vi "PicoScope5000aGetRapidBlockBulk.vi"(0 "handle in":i16, 1 "Rapid Block Acquisition Settings":T4, 2 "Buffer and Transfer Settings":T3 {"Down-Sample Mode" items=["None", "Aggregate", "Decimate", "Average"]; "Down Sample Ratio" step=1}, 7 "enabled array":i16[](array[numeric]), 11 "error in":errorcluster) -> (4 "handle out":i16, 6 "Buffers (Max or non-aggregated)":T2, 8 "Min Buffers":T1, 12 "Num samples":u32, 13 "overflow":i16[](array[numeric]) format="%06b", 15 "error out":errorcluster)   [LabVIEW 2009]
doc: "This VI gets a set of blocks captured using rapid block mode. It outputs max and min clusters with two-dimensional arrays for each channel that contain data from all the requested captures."
uses:
  ps5000a.dll
panel:
  in  "Device Info":T5
  # "Bit 0 = ChA"
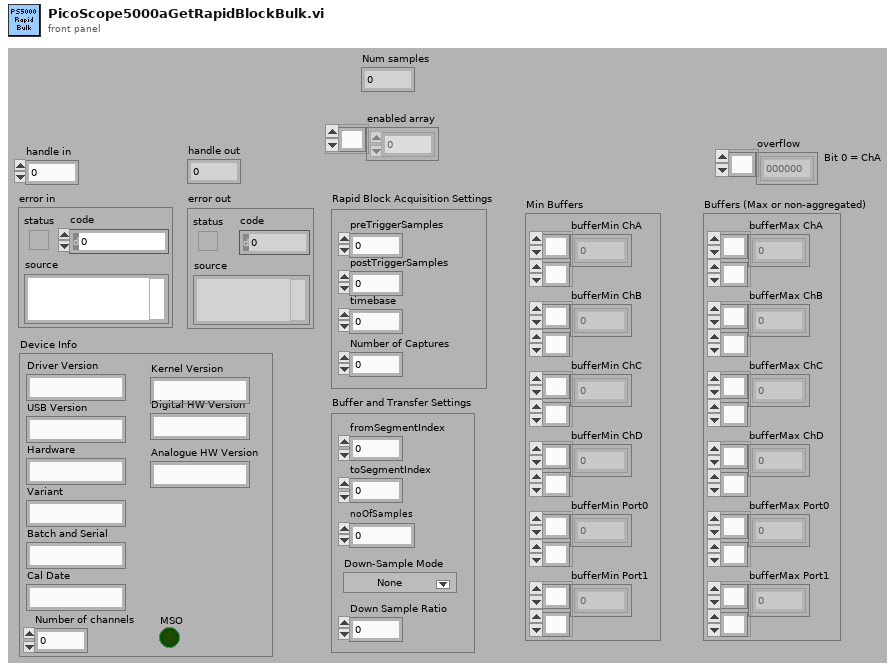
[diagram p1: front panel]
types:
  T1 = cluster{"bufferMin ChA":i16[][], "bufferMin ChB":i16[][], "bufferMin ChC":i16[][], "bufferMin ChD":i16[][], "bufferMin Port0":i16[][], "bufferMin Port1":i16[][]}
  T2 = cluster{"bufferMax ChA":i16[][], "bufferMax ChB":i16[][], "bufferMax ChC":i16[][], "bufferMax ChD":i16[][], "bufferMax Port0":i16[][], "bufferMax Port1":i16[][]}
  T3 = cluster{"fromSegmentIndex":u32, "toSegmentIndex":u32, "noOfSamples":u32, "Down-Sample Mode":u32, "Down Sample Ratio":u32}
  T4 = cluster{"preTriggerSamples":u32, "postTriggerSamples":u32, "timebase":u32, "Number of Captures":u32}
  T5 = cluster{"Driver Version":string, "USB Version":string, "Hardware":string, "Variant":string, "Batch and Serial":string, "Cal Date":string, "Kernel Version":string, "Digital HW Version":string, "Analogue HW Version":string, "MSO":bool, "Number of channels":i16}
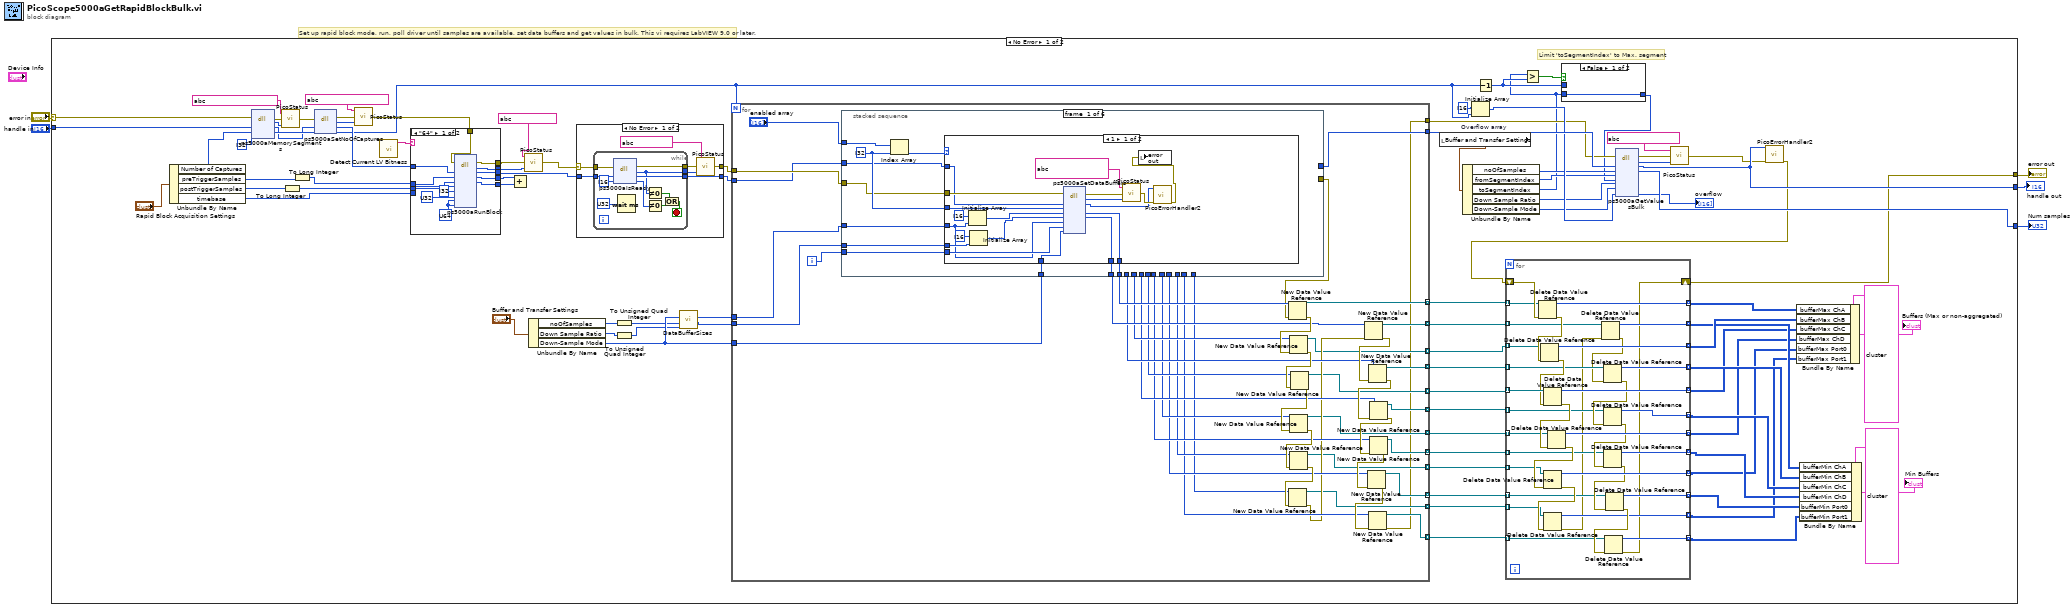
[diagram p0: block diagram]
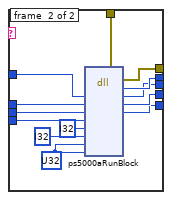
[diagram p3: hidden frame]
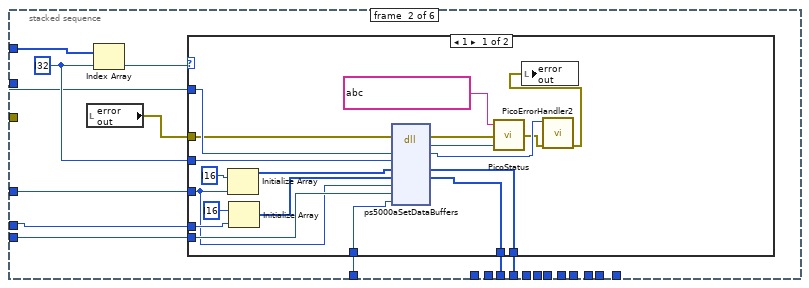
[diagram p5: hidden frame]
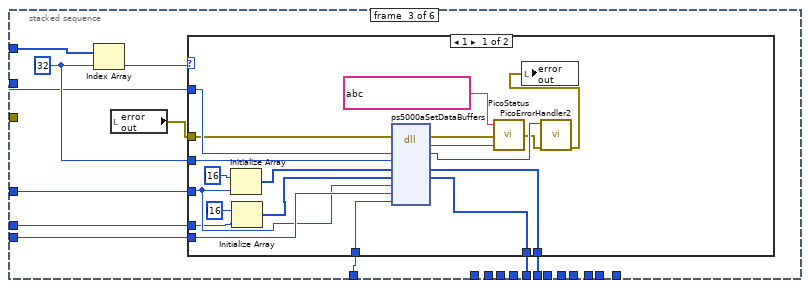
[diagram p7: hidden frame]
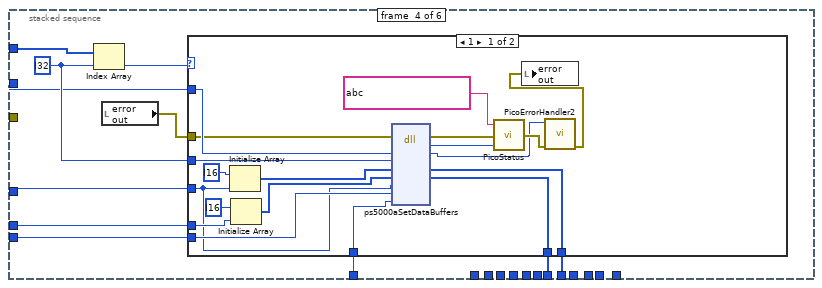
[diagram p9: hidden frame]
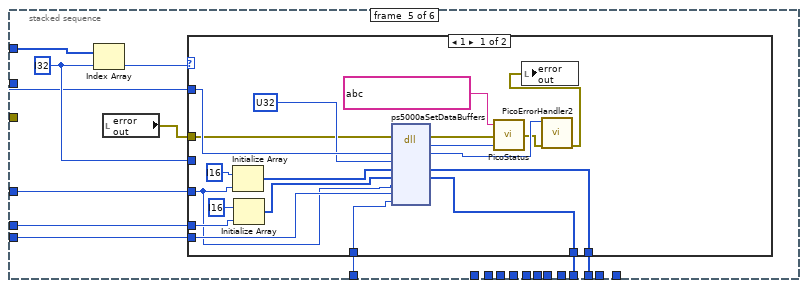
[diagram p11: hidden frame]
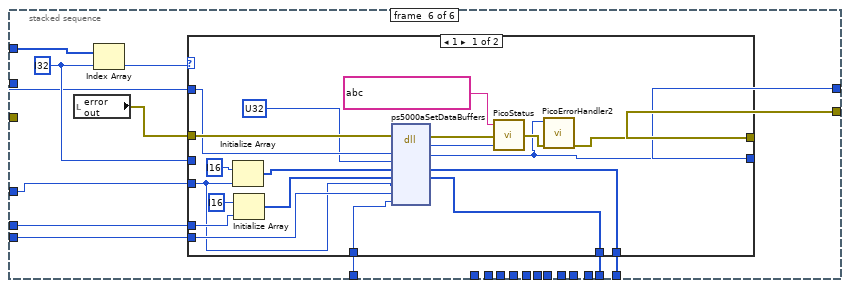
[diagram p13: hidden frame]
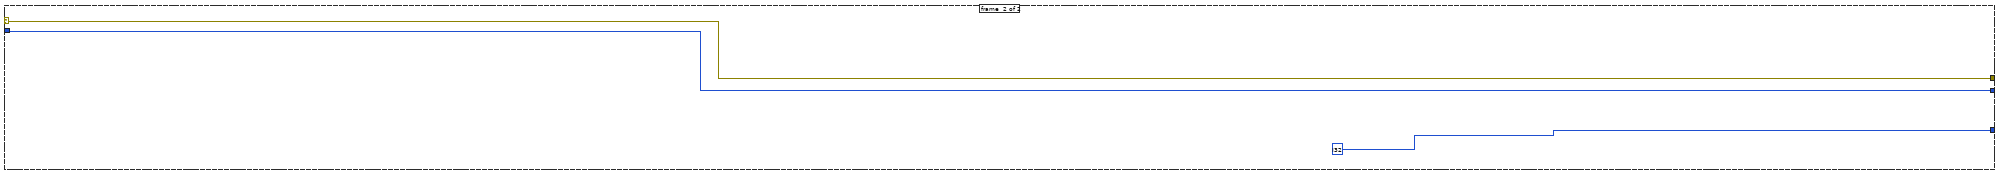
[diagram p16: hidden frame]
diagram:
  # "Set up rapid block mode, run, poll driver until samples are available, set data buffers and get values in bulk. This vi requires LabVIEW 9.0 or later."
  n1 = case shown="No Error" "error in" {
    selector: "error in" -> [w89 w412]
    tunnel: [w21 w412] -> w1
    tunnel: "handle in" -> [w88 w411]
    tunnel: [w68 w411] -> w3
    tunnel: [w69 i32 ?] -> w2
    frame #0 {
      # "Limit 'toSegmentIndex' to Max. segment"
      n2 = Unbundle By Name("Rapid Block Acquisition Settings") -> ("Number of Captures"=w84:u32, "preTriggerSamples"=w66:u32, "postTriggerSamples"=w64:u32, "timebase"=w93:u32)
      n3 = dll-call lib="ps5000a.dll" fn="ps5000aMemorySegments" ("ps3000.dll:_ps3000_open_unit@0")(error in=w89, "handle"=w88, "nSegments"=w84, "nMaxSamples"=i32 ?) -> (error out=w86:errorcluster, "PICO_STATUS"=w87:u32, "handle"=w81:i16, "nSegments"=w82:u32)  [unwired: 3 in, 1 out]
      n4 = call "PicoStatus.vi"("PICO STATUS"=w87, "error in"=w86, "source"=string ?) -> ("error out"=w80:errorcluster)
      n5 = To Long Integer(number=w64) -> (32bit integer=w63:i32)
      n6 = To Long Integer(number=w66) -> (32bit integer=w65:i32)
      n7 = dll-call lib="ps5000a.dll" fn="ps5000aSetNoOfCaptures" ("ps3000.dll:_ps3000_open_unit@0")(error in=w80, "handle"=w81, "nCaptures"=w82) -> (error out=w78:errorcluster, "PICO_STATUS"=w79:u32, "handle"=w75:i16, "nCaptures"=w12:u32)  [unwired: 2 in, 1 out]
      n8 = call "PicoStatus.vi"("PICO STATUS"=w79, "error in"=w78, "source"=string ?) -> ("error out"=w76:errorcluster)
      n9 = call "Detect Current LV Bitness.vi"() -> ("bitness"=w62:string)  [unwired: 11 in]
      n10 = case shown="\"64\"" w62 {
        tunnel: w93 -> [w143 w160]
        tunnel: [w140 w159] -> w92
        tunnel: w76 -> [w147 w158]
        tunnel: w75 -> [w146 w157]
        tunnel: w65 -> [w145 w156]
        tunnel: w63 -> [w144 w155]
        tunnel: [w139 w154] -> w61
        tunnel: [w138 w153] -> w60
        tunnel: [w137 w152] -> w59
        tunnel: [w136 w151] -> w58
        frame #0 {
          w141 = u64 ? ("lpReady")
          n11 = dll-call lib="ps5000a.dll" fn="ps5000aRunBlock" ("ps3000.dll:_ps3000_open_unit@0")(error in=w147, "handle"=w146, "preTriggerSamples"=w145, "postTriggerSamples"=w144, "timebase"=w143, "timeindisposedMs"=i32 ?, "segmentIndex"=u32 ?, "lpReady"=w141, "pParameter"=w141) -> (error out=w140:errorcluster, "PICO_STATUS"=w139:u32, "handle"=w138:i16, "preTriggerSamples"=w137:i32, "postTriggerSamples"=w136:i32)  [unwired: 7 in, 1 out]
        }
        frame #1 {
          w150 = u32 ? ("pParameter")
          n12 = dll-call lib="ps5000a.dll" fn="ps5000aRunBlock" ("ps3000.dll:_ps3000_open_unit@0")(error in=w158, "handle"=w157, "preTriggerSamples"=w156, "postTriggerSamples"=w155, "timebase"=w160, "timeindisposedMs"=i32 ?, "segmentIndex"=i32 ?, "lpReady"=w150, "pParameter"=w150) -> (error out=w159:errorcluster, "PICO_STATUS"=w154:u32, "handle"=w153:i16, "preTriggerSamples"=w152:i32, "postTriggerSamples"=w151:i32)  [unwired: 7 in, 1 out]
        }
      }
      n13 = Add(x=w59, y=w58) -> ()  [unwired: 1 out]
      n14 = call "PicoStatus.vi"("PICO STATUS"=w61, "error in"=w92, "source"=string ?) -> ("error out"=w91:errorcluster)
      n15 = Unbundle By Name("Buffer and Transfer Settings") -> ("noOfSamples"=w9:u32, "Down Sample Ratio"=w7:u32, "Down-Sample Mode"=w55:u32)
      n16 = case shown="No Error" w91 {
        selector: w91 -> [w394 w408]
        tunnel: w60 -> [w396 w409]
        tunnel: [w395 w409] -> w95
        tunnel: [w393 w408] -> w94
        frame #0 {
          n17 = while {
            tunnel: [w407] -> w395
            tunnel: w396 -> [w406]
            tunnel: [w401] -> w391
            tunnel: w394 -> [w400]
            tunnel: [w399] -> w392
            stop <- w405 stop-if-true
            n18 = dll-call lib="ps5000a.dll" fn="ps5000aIsReady" ("ps3000.dll:_ps3000_open_unit@0")(error in=w400, "handle"=w406, "ready"=i16 ?) -> (error out=w399:errorcluster, "PICO_STATUS"=w401:u32, "handle"=w407:i16, "ready"=w402:i16)  [unwired: 2 in, 1 out]
            n19 = Wait (ms)(milliseconds to wait=u32 ? ("ready")) -> ()  [unwired: 1 out]
            n20 = Not Equal To 0?(x=w401) -> (x != 0?=w403:bool)
            n21 = Not Equal To 0?(x=w402) -> (x != 0?=w404:bool)
            n22 = Or(x=w403, y=w404) -> (x .or. y?=w405:bool)
          }
          n23 = call "PicoStatus.vi"("PICO STATUS"=w391, "error in"=w392, "source"=string ?) -> ("error out"=w393:errorcluster)
        }
        frame #1 {
        }
      }
      n24 = To Unsigned Quad Integer(1:w9) -> (0:w8:u64)
      n25 = To Unsigned Quad Integer(1:w7) -> (0:w6:u64)
      n26 = call "DataBufferSizes.vi"("Down Sample Ratio"=w6, "Number of Samples"=w8, "Down-Sample Mode"=w55) -> ("min Buffer Size"=w56:i32, "Max Buffer Size"=w57:i32)  [unwired: 7 in]
      n27 = for {
        N: w12 -> [_]
        tunnel: w95 -> [w202]
        tunnel: w94 -> [w204]
        tunnel: [w203] -> w71
        tunnel: w57 -> [w201]
        tunnel: w56 -> [w200]
        tunnel: w55 -> [w198]
        tunnel: [w173] -> w52 mode=indexing
        tunnel: [w172] -> w51 mode=indexing
        tunnel: [w171] -> w50 mode=indexing
        tunnel: [w170] -> w49 mode=indexing
        tunnel: [w169] -> w48 mode=indexing
        tunnel: [w168] -> w47 mode=indexing
        tunnel: [w167] -> w46 mode=indexing
        tunnel: [w166] -> w45 mode=indexing
        tunnel: [w165] -> w44 mode=indexing
        tunnel: [w164] -> w43 mode=indexing
        tunnel: [w163] -> w42 mode=indexing
        tunnel: [w162] -> w41 mode=indexing
        tunnel: [w161] -> w15
        i -> [w199]
        n28 = stacked-sequence {
          tunnel: "enabled array" -> [w215 w245 w275 w305 w335 w367]
          tunnel: w204 -> [w213 _ _ _ _ _]
          tunnel: w202 -> [w207 w243 w273 w303 w333 w365]
          tunnel: [w212 _ _ _ _ _] -> w187
          tunnel: [_ _ _ _ _ w363] -> w175
          tunnel: [_ _ _ _ _ w362] -> w203
          tunnel: w199 -> [w208 w242 w272 w302 w332 w364]
          tunnel: w198 -> [w211 w236 w267 w296 w326 w356]
          tunnel: w201 -> [w210 w241 w271 w301 w331 w360]
          tunnel: w200 -> [w209 w240 w266 w300 w330 w359]
          tunnel: [w206 _ _ _ _ _] -> w186
          tunnel: [_ w238 _ _ _ _] -> w185
          tunnel: [_ w237 _ _ _ _] -> w184
          tunnel: [_ _ w269 _ _ _] -> w183
          tunnel: [_ _ w268 _ _ _] -> w182
          tunnel: [_ _ _ w298 _ _] -> w181
          tunnel: [_ _ _ w297 _ _] -> w180
          tunnel: [_ _ _ _ w328 _] -> w179
          tunnel: [_ _ _ _ w327 _] -> w178
          tunnel: [_ _ _ _ _ w358] -> w177
          tunnel: [_ _ _ _ _ w357] -> w176
          frame #0 {
            w216 = i32 ? ("dimension size")
            n29 = Index Array(array=w215, index=w216) -> (element=w214:i16)
            n30 = case shown="1" w214 {
              tunnel: w216 -> [w232 _]
              tunnel: w213 -> [w234 _]
              tunnel: w207 -> [w233 _]
              tunnel: [w218 _] -> w212
              tunnel: w208 -> [w231 _]
              tunnel: w211 -> [w225 _]
              tunnel: w210 -> [w219 _]
              tunnel: w209 -> [w220 _]
              tunnel: [w217 _] -> w206
              frame #0 {
                n31 = Initialize Array(i16 ? ("element"), w219) -> (w222:i16[])
                n32 = Initialize Array(i16 ? ("element"), w220) -> (w221:i16[])
                n33 = dll-call lib="ps5000a.dll" fn="ps5000aSetDataBuffers" ("ps3000.dll:_ps3000_open_unit@0")(error in=w234, "handle"=w233, "channel"=w232, "bufferMax"=w222, "bufferMin"=w221, "bufferLth"=w219, "segmentIndex"=w231, "downSampleRatioMode"=w225) -> (error out=w230:errorcluster, "PICO_STATUS"=w227:u32, "handle"=w226:i16, "bufferMax"=w217:i16[], "bufferMin"=w218:i16[])  [unwired: 6 in, 1 out]
                n34 = call "PicoStatus.vi"("PICO STATUS"=w227, "error in"=w230, "source"=string ?) -> ("error out"=w229:errorcluster)
                n35 = call "PicoErrorHandler2.vi"("error in (no error)"=w229, "handle In"=w226) -> ("error out"=w228:errorcluster)  [unwired: 9 in]
                n36 = local write "error out"(w228) -> ()
              }
              frame #1 {
              }
            }
          }
          frame #1 {
            w246 = i32 ? ("dimension size")
            n37 = local read "error out"() -> (w239:errorcluster)
            n38 = Index Array(array=w245, index=w246) -> (element=w244:i16)
            n39 = case shown="1" w244 {
              tunnel: w246 -> [w263 _]
              tunnel: w243 -> [w264 _]
              tunnel: w242 -> [w262 _]
              tunnel: w241 -> [w251 _]
              tunnel: w240 -> [w253 _]
              tunnel: w239 -> [w250 _]
              tunnel: [w249 _] -> w238
              tunnel: [w248 _] -> w237
              tunnel: w236 -> [w247 _]
              frame #0 {
                n40 = Initialize Array(i16 ? ("element"), w251) -> (w254:i16[])
                n41 = Initialize Array(i16 ? ("element"), w253) -> (w252:i16[])
                n42 = dll-call lib="ps5000a.dll" fn="ps5000aSetDataBuffers" ("ps3000.dll:_ps3000_open_unit@0")(error in=w250, "handle"=w264, "channel"=w263, "bufferMax"=w254, "bufferMin"=w252, "bufferLth"=w251, "segmentIndex"=w262, "downSampleRatioMode"=w247) -> (error out=w261:errorcluster, "PICO_STATUS"=w260:u32, "handle"=w258:i16, "bufferMax"=w248:i16[], "bufferMin"=w249:i16[])  [unwired: 6 in, 1 out]
                n43 = call "PicoStatus.vi"("PICO STATUS"=w260, "error in"=w261, "source"=string ?) -> ("error out"=w257:errorcluster)
                n44 = call "PicoErrorHandler2.vi"("error in (no error)"=w257, "handle In"=w258) -> ("error out"=w259:errorcluster)  [unwired: 9 in]
                n45 = local write "error out"(w259) -> ()
              }
              frame #1 {
              }
            }
          }
          frame #2 {
            w276 = i32 ? ("dimension size")
            n46 = Index Array(array=w275, index=w276) -> (element=w274:i16)
            n47 = local read "error out"() -> (w270:errorcluster)
            n48 = case shown="1" w274 {
              tunnel: w276 -> [w293 _]
              tunnel: w273 -> [w294 _]
              tunnel: w272 -> [w292 _]
              tunnel: w271 -> [w282 _]
              tunnel: w270 -> [w281 _]
              tunnel: [w280 _] -> w269
              tunnel: [w279 _] -> w268
              tunnel: w267 -> [w278 _]
              tunnel: w266 -> [w277 _]
              frame #0 {
                n49 = Initialize Array(i16 ? ("element"), w282) -> (w284:i16[])
                n50 = Initialize Array(i16 ? ("element"), w277) -> (w283:i16[])
                n51 = dll-call lib="ps5000a.dll" fn="ps5000aSetDataBuffers" ("ps3000.dll:_ps3000_open_unit@0")(error in=w281, "handle"=w294, "channel"=w293, "bufferMax"=w284, "bufferMin"=w283, "bufferLth"=w282, "segmentIndex"=w292, "downSampleRatioMode"=w278) -> (error out=w291:errorcluster, "PICO_STATUS"=w290:u32, "handle"=w289:i16, "bufferMax"=w279:i16[], "bufferMin"=w280:i16[])  [unwired: 6 in, 1 out]
                n52 = call "PicoStatus.vi"("PICO STATUS"=w290, "error in"=w291, "source"=string ?) -> ("error out"=w288:errorcluster)
                n53 = call "PicoErrorHandler2.vi"("error in (no error)"=w288, "handle In"=w289) -> ("error out"=w287:errorcluster)  [unwired: 9 in]
                n54 = local write "error out"(w287) -> ()
              }
              frame #1 {
              }
            }
          }
          frame #3 {
            w306 = i32 ? ("dimension size")
            n55 = Index Array(array=w305, index=w306) -> (element=w304:i16)
            n56 = local read "error out"() -> (w299:errorcluster)
            n57 = case shown="1" w304 {
              tunnel: w306 -> [w323 _]
              tunnel: w303 -> [w324 _]
              tunnel: w302 -> [w322 _]
              tunnel: w301 -> [w311 _]
              tunnel: w300 -> [w314 _]
              tunnel: w299 -> [w310 _]
              tunnel: [w309 _] -> w298
              tunnel: [w308 _] -> w297
              tunnel: w296 -> [w307 _]
              frame #0 {
                n58 = Initialize Array(i16 ? ("element"), w311) -> (w313:i16[])
                n59 = Initialize Array(i16 ? ("element"), w314) -> (w312:i16[])
                n60 = dll-call lib="ps5000a.dll" fn="ps5000aSetDataBuffers" ("ps3000.dll:_ps3000_open_unit@0")(error in=w310, "handle"=w324, "channel"=w323, "bufferMax"=w313, "bufferMin"=w312, "bufferLth"=w311, "segmentIndex"=w322, "downSampleRatioMode"=w307) -> (error out=w321:errorcluster, "PICO_STATUS"=w320:u32, "handle"=w317:i16, "bufferMax"=w308:i16[], "bufferMin"=w309:i16[])  [unwired: 6 in, 1 out]
                n61 = call "PicoStatus.vi"("PICO STATUS"=w320, "error in"=w321, "source"=string ?) -> ("error out"=w318:errorcluster)
                n62 = call "PicoErrorHandler2.vi"("error in (no error)"=w318, "handle In"=w317) -> ("error out"=w319:errorcluster)  [unwired: 9 in]
                n63 = local write "error out"(w319) -> ()
              }
              frame #1 {
              }
            }
          }
          frame #4 {
            w336 = i32 ? ("dimension size")
            n64 = Index Array(array=w335, index=w336) -> (element=w334:i16)
            n65 = local read "error out"() -> (w329:errorcluster)
            n66 = case shown="1" w334 {
              tunnel: w336 -> [_ _]
              tunnel: w333 -> [w354 _]
              tunnel: w332 -> [w353 _]
              tunnel: w331 -> [w341 _]
              tunnel: w330 -> [w344 _]
              tunnel: w329 -> [w340 _]
              tunnel: [w339 _] -> w328
              tunnel: [w338 _] -> w327
              tunnel: w326 -> [w337 _]
              frame #0 {
                n67 = Initialize Array(i16 ? ("element"), w341) -> (w343:i16[])
                n68 = Initialize Array(i16 ? ("element"), w344) -> (w342:i16[])
                n69 = dll-call lib="ps5000a.dll" fn="ps5000aSetDataBuffers" ("ps3000.dll:_ps3000_open_unit@0")(error in=w340, "handle"=w354, "channel"=u32 ?, "bufferMax"=w343, "bufferMin"=w342, "bufferLth"=w341, "segmentIndex"=w353, "downSampleRatioMode"=w337) -> (error out=w352:errorcluster, "PICO_STATUS"=w351:u32, "handle"=w349:i16, "bufferMax"=w338:i16[], "bufferMin"=w339:i16[])  [unwired: 6 in, 1 out]
                n70 = call "PicoStatus.vi"("PICO STATUS"=w351, "error in"=w352, "source"=string ?) -> ("error out"=w348:errorcluster)
                n71 = call "PicoErrorHandler2.vi"("error in (no error)"=w348, "handle In"=w349) -> ("error out"=w347:errorcluster)  [unwired: 9 in]
                n72 = local write "error out"(w347) -> ()
              }
              frame #1 {
              }
            }
          }
          frame #5 {
            w368 = i32 ? ("dimension size")
            n73 = local read "error out"() -> (w361:errorcluster)
            n74 = Index Array(array=w367, index=w368) -> (element=w366:i16)
            n75 = case shown="1" w366 {
              tunnel: w368 -> [_ _]
              tunnel: w361 -> [w386 w388]
              tunnel: w365 -> [w385 w389]
              tunnel: w364 -> [w384 _]
              tunnel: [w380 w388] -> w363
              tunnel: [w378 w389] -> w362
              tunnel: w360 -> [w372 _]
              tunnel: w359 -> [w375 _]
              tunnel: [w371 _] -> w358
              tunnel: [w370 _] -> w357
              tunnel: w356 -> [w369 _]
              frame #0 {
                n76 = Initialize Array(i16 ? ("element"), w372) -> (w374:i16[])
                n77 = Initialize Array(i16 ? ("element"), w375) -> (w373:i16[])
                n78 = dll-call lib="ps5000a.dll" fn="ps5000aSetDataBuffers" ("ps3000.dll:_ps3000_open_unit@0")(error in=w386, "handle"=w385, "channel"=u32 ?, "bufferMax"=w374, "bufferMin"=w373, "bufferLth"=w372, "segmentIndex"=w384, "downSampleRatioMode"=w369) -> (error out=w383:errorcluster, "PICO_STATUS"=w382:u32, "handle"=w378:i16, "bufferMax"=w370:i16[], "bufferMin"=w371:i16[])  [unwired: 6 in, 1 out]
                n79 = call "PicoStatus.vi"("PICO STATUS"=w382, "error in"=w383, "source"=string ?) -> ("error out"=w379:errorcluster)
                n80 = call "PicoErrorHandler2.vi"("error in (no error)"=w379, "handle In"=w378) -> ("error out"=w380:errorcluster)  [unwired: 9 in]
              }
              frame #1 {
              }
            }
          }
        }
        n81 = New Data Value Reference(data value=w186, error in=w175) -> (data value reference=w173:refnum<data-value>, error out=w194:errorcluster)
        n82 = New Data Value Reference(data value=w184, error in=w194) -> (data value reference=w171:refnum<data-value>, error out=w193:errorcluster)
        n83 = New Data Value Reference(data value=w182, error in=w193) -> (data value reference=w166:refnum<data-value>, error out=w197:errorcluster)
        n84 = New Data Value Reference(data value=w180, error in=w197) -> (data value reference=w168:refnum<data-value>, error out=w196:errorcluster)
        n85 = New Data Value Reference(data value=w178, error in=w196) -> (data value reference=w165:refnum<data-value>, error out=w195:errorcluster)
        n86 = New Data Value Reference(data value=w176, error in=w195) -> (data value reference=w163:refnum<data-value>, error out=w174:errorcluster)
        n87 = New Data Value Reference(data value=w187, error in=w174) -> (data value reference=w172:refnum<data-value>, error out=w189:errorcluster)
        n88 = New Data Value Reference(data value=w185, error in=w189) -> (data value reference=w170:refnum<data-value>, error out=w188:errorcluster)
        n89 = New Data Value Reference(data value=w183, error in=w188) -> (data value reference=w169:refnum<data-value>, error out=w192:errorcluster)
        n90 = New Data Value Reference(data value=w181, error in=w192) -> (data value reference=w167:refnum<data-value>, error out=w191:errorcluster)
        n91 = New Data Value Reference(data value=w179, error in=w191) -> (data value reference=w164:refnum<data-value>, error out=w190:errorcluster)
        n92 = New Data Value Reference(data value=w177, error in=w190) -> (data value reference=w162:refnum<data-value>, error out=w161:errorcluster)
      }
      n93 = local read "Buffer and Transfer Settings"() -> (w20:T3)
      n94 = Unbundle By Name(w20) -> ("noOfSamples"=w16:u32, "fromSegmentIndex"=w17:u32, "toSegmentIndex"=w11:u32, "Down Sample Ratio"=w18:u32, "Down-Sample Mode"=w19:u32)
      n95 = Initialize Array "Overflow array"(i16 ? ("element"), w12) -> (w53:i16[])
      n96 = Decrement(x=w12) -> (x-1=w14:u32)
      n97 = Greater?(x=w11, y=w14) -> (0:w13:bool)
      n98 = case shown="False" w13 {
        tunnel: [w96 w97] -> w10
        tunnel: w11 -> [w96 _]
        tunnel: w14 -> [_ w97]
        frame #0 {
        }
        frame #1 {
        }
      }
      n99 = dll-call lib="ps5000a.dll" fn="ps5000aGetValuesBulk" ("ps3000.dll:_ps3000_open_unit@0")(error in=w15, "handle"=w71, "noOfSamples"=w16, "fromSegmentIndex"=w17, "toSegmentIndex"=w10, "downSampleRatio"=w18, "downSampleRatioMode"=w19, "overflow"=w53) -> (error out=w73:errorcluster, "PICO_STATUS"=w72:u32, "handle"=w68:i16, "noOfSamples"=w69:u32, "overflow"=→"overflow":i16[])  [unwired: 6 in, 1 out]
      n100 = call "PicoStatus.vi"("PICO STATUS"=w72, "error in"=w73, "source"=string ?) -> ("error out"=w23:errorcluster)
      n101 = call "PicoErrorHandler2.vi"("error in (no error)"=w23, "handle In"=w68) -> ("error out"=w22:errorcluster)  [unwired: 9 in]
      n102 = for {
        shift-right: [w98] -> w21
        shift-left: w22 -> [w127]
        tunnel: w45 -> [w134] mode=indexing
        tunnel: [w130] -> w28 mode=indexing
        tunnel: [w129] -> w27 mode=indexing
        tunnel: [w128] -> w26 mode=indexing
        tunnel: w50 -> [w124] mode=indexing
        tunnel: w52 -> [w123] mode=indexing
        tunnel: [w122] -> w35 mode=indexing
        tunnel: [w121] -> w36 mode=indexing
        tunnel: w51 -> [w120] mode=indexing
        tunnel: w49 -> [w119] mode=indexing
        tunnel: w48 -> [w116] mode=indexing
        tunnel: w47 -> [w115] mode=indexing
        tunnel: w46 -> [w111] mode=indexing
        tunnel: w44 -> [w110] mode=indexing
        tunnel: w43 -> [w109] mode=indexing
        tunnel: w42 -> [w108] mode=indexing
        tunnel: w41 -> [w107] mode=indexing
        tunnel: [w106] -> w34 mode=indexing
        tunnel: [w105] -> w33 mode=indexing
        tunnel: [w104] -> w32 mode=indexing
        tunnel: [w103] -> w31 mode=indexing
        tunnel: [w102] -> w30 mode=indexing
        tunnel: [w101] -> w29 mode=indexing
        tunnel: [w100] -> w25 mode=indexing
        n103 = Delete Data Value Reference(data value reference=w123, error in=w127) -> (data value=w121:i16[], error out=w126:errorcluster)
        n104 = Delete Data Value Reference(data value reference=w124, error in=w126) -> (data value=w122:i16[], error out=w125:errorcluster)
        n105 = Delete Data Value Reference(data value reference=w134, error in=w125) -> (data value=w130:i16[], error out=w133:errorcluster)
        n106 = Delete Data Value Reference(data value reference=w115, error in=w133) -> (data value=w129:i16[], error out=w132:errorcluster)
        n107 = Delete Data Value Reference(data value reference=w110, error in=w132) -> (data value=w128:i16[], error out=w131:errorcluster)
        n108 = Delete Data Value Reference(data value reference=w108, error in=w131) -> (data value=w100:i16[], error out=w99:errorcluster)
        n109 = Delete Data Value Reference(data value reference=w120, error in=w99) -> (data value=w106:i16[], error out=w118:errorcluster)
        n110 = Delete Data Value Reference(data value reference=w119, error in=w118) -> (data value=w105:i16[], error out=w117:errorcluster)
        n111 = Delete Data Value Reference(data value reference=w116, error in=w117) -> (data value=w104:i16[], error out=w112:errorcluster)
        n112 = Delete Data Value Reference(data value reference=w111, error in=w112) -> (data value=w103:i16[], error out=w114:errorcluster)
        n113 = Delete Data Value Reference(data value reference=w109, error in=w114) -> (data value=w102:i16[], error out=w113:errorcluster)
        n114 = Delete Data Value Reference(data value reference=w107, error in=w113) -> (data value=w101:i16[], error out=w98:errorcluster)
      }
      n115 = Bundle By Name(cluster=T2 ?, "bufferMax ChA"=w36, "bufferMax ChB"=w35, "bufferMax ChC"=w28, "bufferMax ChD"=w27, "bufferMax Port0"=w26, "bufferMax Port1"=w25) -> (→"Buffers (Max or non-aggregated)":T2)
      n116 = Bundle By Name(cluster=T1 ? ("Min Buffers 2"), "bufferMin ChA"=w34, "bufferMin ChB"=w33, "bufferMin ChC"=w32, "bufferMin ChD"=w31, "bufferMin Port0"=w30, "bufferMin Port1"=w29) -> (→"Min Buffers":T1)
    }
    frame #1 {
    }
  }
  "handle out" <- w3
  "Num samples" <- w2
  "error out" <- w1
